vi "DescribeTextField.vi"(0 "XRef":T21, 1 "ID":T3, 2 "State In":T14) -> (14 "Text Field Info":T2, 15 "Fatal Error Out":T1)   [LabVIEW 2020, in "Parallel Diagram Block.xnode"]
uses:
  Parallel Diagram Block.xnode
  <vilib>/XNodeSupport/XNodeXNodeRef.ctl
  <vilib>/XNodeSupport/XNodeString.ctl
  State.ctl
  Parallel Block/Type Descriptor.ctl
  Parallel Block/Direction.ctl
  Parallel Block/Value Type.ctl
  Parallel Block/Terminal Mode.ctl
  Parallel Block/Terminal Type.ctl
  <vilib>/picture/picture.llb/imagedata.ctl
  <vilib>/XNodeSupport/XNodeTextFieldInfo.ctl
  <vilib>/XNodeSupport/XNodeRect32.ctl
  <vilib>/XNodeSupport/XNodeInt.ctl
  <vilib>/XNodeSupport/XNodeJustification.ctl
  <vilib>/XNodeSupport/XNodeHorizontal.ctl
  <vilib>/XNodeSupport/XNodeVertical.ctl
  <vilib>/XNodeSupport/XNodeColor.ctl
  <vilib>/XNodeSupport/XNodeFont.ctl
  <vilib>/XNodeSupport/XNodeUserFont.ctl
  <vilib>/XNodeSupport/XNodeUInt.ctl
  <vilib>/XNodeSupport/XNodeBool.ctl
  <vilib>/XNodeSupport/XNodeErrorCluster.ctl
  <vilib>/XNodeSupport/NI_XNodeSupport.lvlib
  Parallel Block/Parallel Block.lvlib
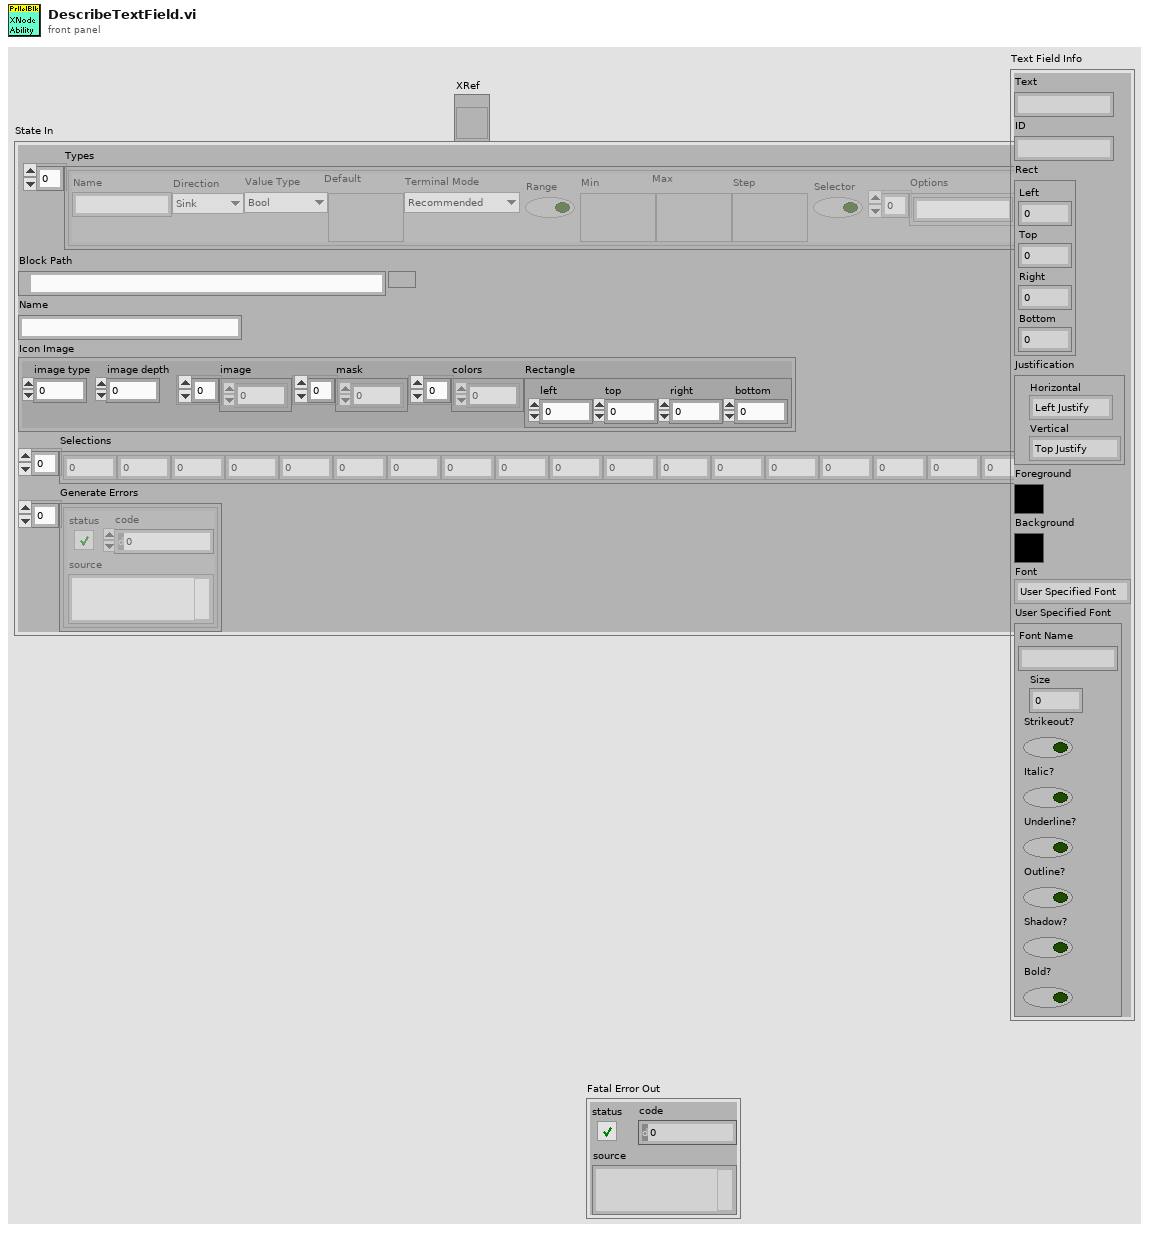
[diagram p1: front panel]
types:
  T1 = typedef "NI_XNodeSupport.lvlib/XNodeErrorCluster.ctl" = errorcluster
  T2 = typedef "NI_XNodeSupport.lvlib/XNodeTextFieldInfo.ctl" = cluster{"Text":T3, "ID":T3, "Rect":T4, "Justification":T6, "Foreground":T9, "Background":T9, "Font":T10, "User Specified Font":T11}
  T3 = typedef "NI_XNodeSupport.lvlib/XNodeString.ctl" = string
  T4 = typedef "NI_XNodeSupport.lvlib/XNodeRect32.ctl" = cluster{"Left":T5, "Top":T5, "Right":T5, "Bottom":T5}
  T5 = typedef "NI_XNodeSupport.lvlib/XNodeInt.ctl" = i32
  T6 = typedef "NI_XNodeSupport.lvlib/XNodeJustification.ctl" = cluster{"Horizontal":T7, "Vertical":T8}
  T7 = typedef "NI_XNodeSupport.lvlib/XNodeHorizontal.ctl" = enum32{"Left Justify", "Right Justify", "CenterJustify"}
  T8 = typedef "NI_XNodeSupport.lvlib/XNodeVertical.ctl" = enum32{"Top Justify", "Bottom Justify", "CenterJustify"}
  T9 = typedef "NI_XNodeSupport.lvlib/XNodeColor.ctl" = u32
  T10 = typedef "NI_XNodeSupport.lvlib/XNodeFont.ctl" = enum32{"User Specified Font", "Application Font", "System Font", "Dialog Font"}
  T11 = typedef "NI_XNodeSupport.lvlib/XNodeUserFont.ctl" = cluster{"Font Name":T3, "Size":T12, "Strikeout?":T13, "Italic?":T13, "Underline?":T13, "Outline?":T13, "Shadow?":T13, "Bold?":T13}
  T12 = typedef "NI_XNodeSupport.lvlib/XNodeUInt.ctl" = u32
  T13 = typedef "NI_XNodeSupport.lvlib/XNodeBool.ctl" = bool
  T14 = typedef "Parallel Diagram Block.xnode/State.ctl" = cluster{"Types":T15[], "Block Path":path, "Name":string, "Icon Image":T20, "Selections":i32[], "Generate Errors":errorcluster[]}
  T15 = typedef "Parallel Block.lvlib/Type Descriptor.ctl" = cluster{"Name":string, "Direction":T16, "Value Type":T17, "Default":variant, "Terminal Mode":T18, "Range":bool, "Min":variant, "Max":variant, "Step":variant, "Selector":bool, "Options":string[], "Terminal Type":T19}
  T16 = typedef "Parallel Block.lvlib/Direction.ctl" = enum16{"Sink", "Source"}
  T17 = typedef "Parallel Block.lvlib/Value Type.ctl" = enum16{"Unknown", "Bool", "U8", "U16", "U32", "U64", "I8", "I16", "I32", "I64", "SGL", "DBL", "CSG", "CDB", "CDBWfm", "String", "DBLWfm"}
  T18 = typedef "Parallel Block.lvlib/Terminal Mode.ctl" = enum16{"Recommended", "Required", "None"}
  T19 = typedef "Parallel Block.lvlib/Terminal Type.ctl" = enum16{"Unwired", "BadType", "Connection", "Value", "Control Ref", "BadRefType"}
  T20 = typedef "imagedata.ctl" = cluster{"image type":i32, "image depth":i32, "image":u8[], "mask":u8[], "colors":u32[], "Rectangle":cluster{"left":i16, "top":i16, "right":i16, "bottom":i16}}
  T21 = typedef "NI_XNodeSupport.lvlib/XNodeXNodeRef.ctl" = refnum<vi>
  T22 = cluster{"left":i16, "top":i16, "right":i16, "bottom":i16}
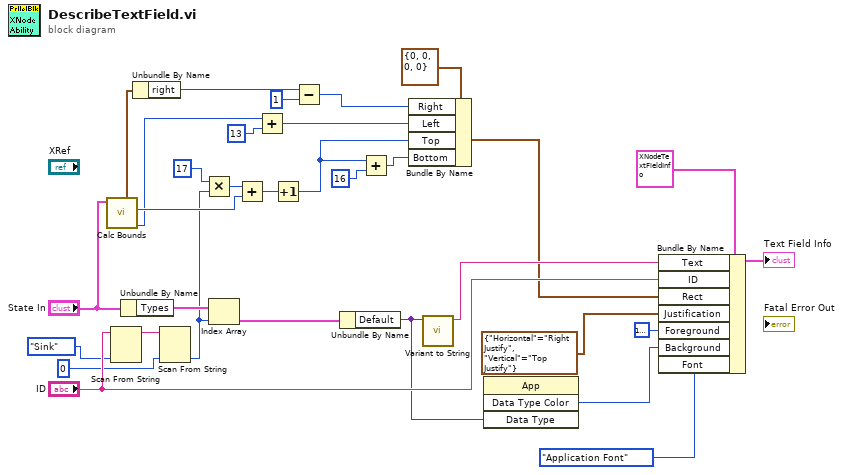
[diagram p0: block diagram]
diagram:
  n1 = call "Calc Bounds.vi"("State"="State In") -> ("Name Width"=w3:i16, "Header"=w17:i32, "Bounds Without Terminals"=w14:T22)  [unwired: 4 in, 4 out]
  n2 = Scan From String(input string="ID", default 1=Direction."Sink" ("Direction")) -> (remaining string=w10:string)  [unwired: 4 in, 2 out]
  n3 = Unbundle By Name("State In") -> ("Types"=w27:T15[])
  n4 = Unbundle By Name(w14) -> ("right"=w6:i16)
  n5 = Scan From String(input string=w10, default 1=0) -> (output 1=w8:i32)  [unwired: 3 in, 3 out]
  n6 = Multiply(x=17, y=w8) -> (x*y=w18:i32)
  n7 = Index Array(array=w27, index=w8) -> (element=w26:T15)
  n8 = Add(x=w18, y=w17) -> (x+y=w13:i32)
  n9 = Add(x=w3, y=i16 13) -> (x+y=w2:i16)
  n10 = Increment(x=w13) -> (x+1=w7:i32)
  n11 = Subtract(x=w6, y=i16 1) -> (x-y=w5:i16)
  n12 = Unbundle By Name(w26) -> ("Default"=w23:variant)
  n13 = Add(x=w7, y=16) -> (x+y=w11:i32)
  n14 = Bundle By Name(cluster=T4 {"Left"=0, "Top"=0, "Right"=0, "Bottom"=0} ("Rect"), "Right"=w5, "Left"=w2, "Top"=w7, "Bottom"=w11) -> (w15:T4)
  n15 = call "Variant to String.vi"("Value"=w23) -> ("String"=w25:string)  [unwired: 10 in]
  n16 = invoke class="App" method="Data Type Color"("Data Type"=w23) -> ("Data Type Color"=w22:u32)  [unwired: 3 in, 3 out]
  n17 = Bundle By Name(cluster=T2 {"Text"="", "ID"="", "Rect"={"Left"=0, "Top"=0, "Right"=0, "Bottom"=0}, "Justification"={"Horizontal"=enum."Left Justify", "Vertical"=enum."Top Justify"}, "Foreground"=0, "Background"=0, "Font"=enum."User Specified Font", "User Specified Font"={"Font Name"="", "Size"=0, "Strikeout?"=FALSE, "Italic?"=FALSE, "Underline?"=FALSE, "Outline?"=FALSE, "Shadow?"=FALSE, "Bold?"=FALSE}} ("Text Field Info"), "Text"=w25, "ID"="ID", "Rect"=w15, "Justification"=T6 {"Horizontal"=enum."Right Justify", "Vertical"=enum."Top Justify"}, "Foreground"=T9 16777215, "Background"=w22, "Font"=XNodeFont."Application Font") -> (→"Text Field Info":T2)
